vi "itemstring to item array.vi"(11 "Item sym string":string[](array[string])) -> (3 "Item sym":i32[](array[numeric])=[37, 37, 38, 38])   [LabVIEW 2012]
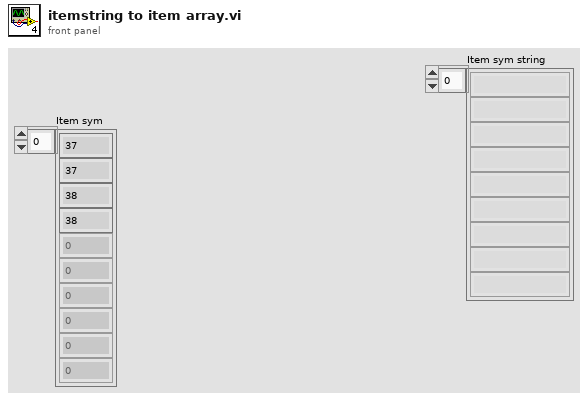
[diagram p1: front panel]
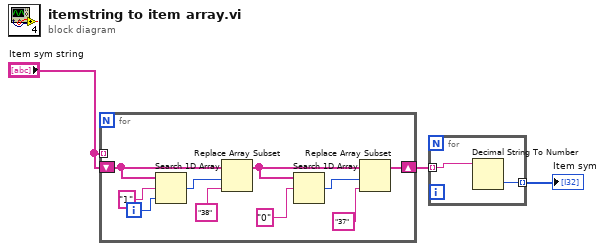
[diagram p0: block diagram]
diagram:
  n1 = for {
    tunnel: "Item sym string" -> [_] mode=indexing
    shift-right: [w9] -> w3
    shift-left: "Item sym string" -> [w10]
    i -> [w13]
    n2 = Search 1D Array(1D array=w10, element="1", start index (0)=w13) -> (index of element=w12:i32)
    n3 = Replace Array Subset(array=w10, new element="38", index=w12) -> (w8:string[])
    n4 = Search 1D Array(1D array=w8, element="0") -> (index of element=w11:i32)  [unwired: 1 in]
    n5 = Replace Array Subset(array=w8, new element="37", index=w11) -> (w9:string[])
  }
  n6 = for {
    tunnel: w3 -> [w15] mode=indexing
    tunnel: [w14] -> w1 mode=indexing
    n7 = Decimal String To Number(string=w15) -> (number=w14:i32)  [unwired: 2 in, 1 out]
  }
  "Item sym" <- w1
